vi "S4GUI_001.vi"() -> ()   [LabVIEW 2018] (continued)
                n1368 = call-dynamic "Write Channel.vi"("error in (no error)"=w2937, "Channel.lvclass"=w2938, "Acquisition in"=w2967) -> ("error out"=w2933:errorcluster, "Acquisition out"=w2934:refnum<class "Acquisition.lvclass">)  [unwired: 7 in]
              }
            }
            n1369 = case shown="True" w2918 {
              tunnel: w2920 -> [w3009 w3014]
              tunnel: w2919 -> [w3008 w3013]
              tunnel: [w3009 w3012] -> w2889
              tunnel: [w3008 w3011] -> w2888
              tunnel: w2882 -> [_ w3010]
              frame False {
              }
              frame True {
                # "nome do arquivo .cfg"
                # "seção no arquivo .cfg"
                n1370 = call-dynamic "Read Channel.vi"("error in (no error)"=w3013, "Acquisition in"=w3014) -> ("error out"=w3018:errorcluster, "Channel.lvclass"=w3017:refnum<class "Channel.lvclass">, "Acquisition out"=w3016:refnum<class "Acquisition.lvclass">)  [unwired: 7 in]
                n1371 = call-dynamic "Read Interface.vi"("error in (no error)"=w3018, "Channel in"=w3017) -> ("error out"=w3025:errorcluster, "Interface.lvclass"=w3026:refnum<class "Interface.lvclass">, "Channel out"=w3015:refnum<class "Channel.lvclass">)  [unwired: 7 in]
                n1372 = call-dynamic "Get CCD_Config.vi"("error in (no error)"=w3025, "Interface in"=w3026) -> ("error out"=w3023:errorcluster, "output cluster"=w3022:T24, "Interface out"=w3027:refnum<class "Interface.lvclass">)  [unwired: 7 in]
                n1373 = Bundle By Name(cluster=w3022, "TRIGGER_MODE"=w3010) -> (w3024:T24)
                n1374 = call-dynamic "Set CCD_Config.vi"("error in (no error)"=w3023, "input cluster"=w3024, "Interface in"=w3027) -> ("error out"=w3021:errorcluster, "Interface out"=w3028:refnum<class "Interface.lvclass">)  [unwired: 7 in]
                n1375 = Flatten To String(anything=w3024, error in (no error)=w3021) -> (data string=w3019:string, error out=w3020:errorcluster)  [unwired: 2 in, 1 out]
                n1376 = call "Write flatted cluster.vi"("error in (no error)"=w3020, "flatted cluster"=w3019, "Interface in"=w3028) -> ("error out"=w3030:errorcluster, "Interface out"=w3029:refnum<class "Interface.lvclass">)  [unwired: 7 in]
                n1377 = call-dynamic "Write Interface.vi"("error in (no error)"=w3030, "Interface.lvclass"=w3029, "Channel in"=w3015) -> ("error out"=w3036:errorcluster, "Channel out"=w3037:refnum<class "Channel.lvclass">)  [unwired: 7 in]
                n1378 = call "Write section_name.vi"("error in (no error)"=w3036, "section_name"="CCD_ACS2", "Channel in"=w3037) -> ("error out"=w3034:errorcluster, "Channel out"=w3040:refnum<class "Channel.lvclass">)  [unwired: 7 in]
                n1379 = call-dynamic "save config.vi"("error in (no error)"=w3034, "file config"="lastsaved.cfg", "Channel in"=w3040) -> ("error out"=w3035:errorcluster, "Channel out"=w3041:refnum<class "Channel.lvclass">)  [unwired: 7 in]
                n1380 = call-dynamic "Read State Machine.vi"("error in (no error)"=w3035, "Device in"=w3041) -> ("error out"=w3031:errorcluster, "State Machine.lvclass"=w3043:refnum<class "State Machine.lvclass">, "Device out"=w3042:refnum<class "Channel.lvclass">)  [unwired: 7 in]
                n1381 = call-dynamic "Write State.vi"("error in (no error)"=w3031, "State"=60, "State Machine in"=w3043) -> ("error out"=w3032:errorcluster, "State Machine out"=w3044:refnum<class "State Machine.lvclass">)  [unwired: 7 in]
                n1382 = call-dynamic "Write State Machine.vi"("error in (no error)"=w3032, "State Machine.lvclass"=w3044, "Device in"=w3042) -> ("error out"=w3046:errorcluster, "Device out"=w3045:refnum<class "Channel.lvclass">)  [unwired: 7 in]
                n1383 = call-dynamic "Write Channel.vi"("error in (no error)"=w3046, "Channel.lvclass"=w3045, "Acquisition in"=w3016) -> ("error out"=w3011:errorcluster, "Acquisition out"=w3012:refnum<class "Acquisition.lvclass">)  [unwired: 7 in]
              }
            }
            n1384 = case shown="True" w2921 {
              tunnel: [w3047 w3081] -> w2890
              tunnel: [w3048 w3080] -> w2891
              tunnel: w2923 -> [w3048 w3051]
              tunnel: w2922 -> [w3047 w3050]
              tunnel: w2882 -> [_ w3049]
              frame False {
              }
              frame True {
                # "nome do arquivo .cfg"
                # "seção no arquivo .cfg"
                n1385 = call-dynamic "Read Channel.vi"("error in (no error)"=w3050, "Acquisition in"=w3051) -> ("error out"=w3082:errorcluster, "Channel.lvclass"=w3083:refnum<class "Channel.lvclass">, "Acquisition out"=w3084:refnum<class "Acquisition.lvclass">)  [unwired: 7 in]
                n1386 = call-dynamic "Read Interface.vi"("error in (no error)"=w3082, "Channel in"=w3083) -> ("error out"=w3073:errorcluster, "Interface.lvclass"=w3072:refnum<class "Interface.lvclass">, "Channel out"=w3085:refnum<class "Channel.lvclass">)  [unwired: 7 in]
                n1387 = call-dynamic "Get CCD_Config.vi"("error in (no error)"=w3073, "Interface in"=w3072) -> ("error out"=w3075:errorcluster, "output cluster"=w3076:T24, "Interface out"=w3071:refnum<class "Interface.lvclass">)  [unwired: 7 in]
                n1388 = Bundle By Name(cluster=w3076, "TRIGGER_MODE"=w3049) -> (w3074:T24)
                n1389 = call-dynamic "Set CCD_Config.vi"("error in (no error)"=w3075, "input cluster"=w3074, "Interface in"=w3071) -> ("error out"=w3077:errorcluster, "Interface out"=w3070:refnum<class "Interface.lvclass">)  [unwired: 7 in]
                n1390 = Flatten To String(anything=w3074, error in (no error)=w3077) -> (data string=w3079:string, error out=w3078:errorcluster)  [unwired: 2 in, 1 out]
                n1391 = call "Write flatted cluster.vi"("error in (no error)"=w3078, "flatted cluster"=w3079, "Interface in"=w3070) -> ("error out"=w3068:errorcluster, "Interface out"=w3069:refnum<class "Interface.lvclass">)  [unwired: 7 in]
                n1392 = call-dynamic "Write Interface.vi"("error in (no error)"=w3068, "Interface.lvclass"=w3069, "Channel in"=w3085) -> ("error out"=w3063:errorcluster, "Channel out"=w3062:refnum<class "Channel.lvclass">)  [unwired: 7 in]
                n1393 = call "Write section_name.vi"("error in (no error)"=w3063, "section_name"="CCD_ACS1", "Channel in"=w3062) -> ("error out"=w3064:errorcluster, "Channel out"=w3059:refnum<class "Channel.lvclass">)  [unwired: 7 in]
                n1394 = call-dynamic "save config.vi"("error in (no error)"=w3064, "file config"="lastsaved.cfg", "Channel in"=w3059) -> ("error out"=w3052:errorcluster, "Channel out"=w3053:refnum<class "Channel.lvclass">)  [unwired: 7 in]
                n1395 = call-dynamic "Read State Machine.vi"("error in (no error)"=w3052, "Device in"=w3053) -> ("error out"=w3067:errorcluster, "State Machine.lvclass"=w3057:refnum<class "State Machine.lvclass">, "Device out"=w3058:refnum<class "Channel.lvclass">)  [unwired: 7 in]
                n1396 = call-dynamic "Write State.vi"("error in (no error)"=w3067, "State"=60, "State Machine in"=w3057) -> ("error out"=w3066:errorcluster, "State Machine out"=w3056:refnum<class "State Machine.lvclass">)  [unwired: 7 in]
                n1397 = call-dynamic "Write State Machine.vi"("error in (no error)"=w3066, "State Machine.lvclass"=w3056, "Device in"=w3058) -> ("error out"=w3054:errorcluster, "Device out"=w3055:refnum<class "Channel.lvclass">)  [unwired: 7 in]
                n1398 = call-dynamic "Write Channel.vi"("error in (no error)"=w3054, "Channel.lvclass"=w3055, "Acquisition in"=w3084) -> ("error out"=w3081:errorcluster, "Acquisition out"=w3080:refnum<class "Acquisition.lvclass">)  [unwired: 7 in]
              }
            }
            n1399 = call-dynamic "Write AcquisitionA.vi"("error in (no error)"=w2890, "Acquisition.lvclass"=w2891, "S4ACS_GUI in"=w2892) -> ("error out"=w2898:errorcluster, "S4ACS_GUI out"=w2901:refnum<class "S4GUI.lvclass">)  [unwired: 7 in]
            n1400 = call "Write AcquisitionB.vi"("error in (no error)"=w2888, "Acquisition.lvclass"=w2889, "S4ACS_GUI in"=w2901) -> ("error out"=w2897:errorcluster, "S4ACS_GUI out"=w2900:refnum<class "S4GUI.lvclass">)  [unwired: 7 in]
            n1401 = call-dynamic "Write AcquisitionC.vi"("error in (no error)"=w2886, "Acquisition.lvclass"=w2887, "S4ACS_GUI in"=w2900) -> ("error out"=w2896:errorcluster, "S4ACS_GUI out"=w2899:refnum<class "S4GUI.lvclass">)  [unwired: 7 in]
            n1402 = call-dynamic "Write AcquisitionD.vi"("error in (no error)"=w2884, "Acquisition.lvclass"=w2885, "S4ACS_GUI in"=w2899) -> ("error out"=w2895:errorcluster, "S4ACS_GUI out"=w2894:refnum<class "S4GUI.lvclass">)  [unwired: 7 in]
            n1403 = Merge Errors(w2898, w2897, w2896, w2895) -> (w2893:errorcluster)
          }
        }
        n1404 = call-dynamic "Write sync.vi"("error in (no error)"=w2669, "sync"=w2672, "S4ACS_GUI in"=w2670) -> ("error out"=w2658:errorcluster, "S4ACS_GUI out"=w2671:refnum<class "S4GUI.lvclass">)  [unwired: 7 in]
      }
      event "ExtSync": Value Change {
        n1405 = event-data() -> ("NewVal"=w3169:bool)  [unwired: 1 in]
        n1406 = Not(x=w3169) -> (.not. x?=w3088:bool)
        n1407 = call-dynamic "Read Sync Box.lvclass.vi"("error in (no error)"=w3172, "SPARC4_AC in"=w3181) -> ("error out"=w3174:errorcluster, "Sync Box.lvclass"=w3180:refnum<class "Sync Box.lvclass">, "SPARC4_AC out"=w3177:refnum<class "S4GUI.lvclass">)  [unwired: 7 in]
        n1408 = call-dynamic "Read Stream.vi"("error in (no error)"=w3174, "Server in"=w3180) -> ("error out"=w3173:errorcluster, "Stream.lvclass"=w3182:refnum<class "Stream.lvclass">, "Server out"=w3171:refnum<class "Sync Box.lvclass">)  [unwired: 7 in]
        n1409 = case shown="True" w3169 {
          tunnel: [w3187 w3204] -> w3175
          tunnel: w3182 -> [w3189 w3192]
          tunnel: [w3188 w3200] -> w3179
          tunnel: w3173 -> [w3185 w3191]
          tunnel: w3171 -> [w3186 w3194]
          tunnel: [w3183 w3193] -> w3170
          frame False {
            n1410 = call-dynamic "ReleaseQueueTCPIP.vi"("error in (no error)"=w3185, "Server in"=w3186) -> ("error out"=w3184:errorcluster, "Server out"=w3183:refnum<class "Sync Box.lvclass">)  [unwired: 8 in]
            n1411 = call-dynamic "End.vi"("error in (no error)"=w3184, "Stream in"=w3189) -> ("error out"=w3187:errorcluster, "Stream out"=w3188:refnum<class "Stream.lvclass">)  [unwired: 8 in]
          }
          frame True {
            w3197 = errorcluster {"status"=FALSE, "code"=0, "source"=""} ("error in (no error)")
            w3216 = FALSE ("Wait Until Done")
            w3211 = FALSE ("Wait Until Done")
            n1412 = call-dynamic "Send TCP Param.vi"("error in (no error)"=w3191, "Server in"=w3194) -> ("error out"=w3190:errorcluster, "Server out"=w3193:refnum<class "Sync Box.lvclass">)  [unwired: 8 in]
            n1413 = call-dynamic "Read StreamRX filename.vi"("error in (no error)"=w3190, "Stream in"=w3192) -> ("error out"=w3207:errorcluster, "StreamRX filename"=w3208:string, "Stream out"=w3203:refnum<class "Stream.lvclass">)  [unwired: 7 in]
            n1414 = call <vilib>:"Application Directory.vi"() -> ("Application Directory"=w3213:path)
            n1415 = call <vilib>:"Application Directory.vi"() -> ("Application Directory"=w3217:path)
            n1416 = Build Path(base path=w3217, name or relative path=w3208) -> (appended path=w3218:path)
            n1417 = Open VI Reference(vi path=w3218, error in (no error)=w3207) -> (vi reference=w3210:refnum<vi>, error out=w3209:errorcluster)  [unwired: 4 in]
            n1418 = invoke class="VI" method="Run VI"(reference=w3210, error in=w3209, "Wait until done"=w3211, "Auto Dispose Ref"=w3211) -> (reference out=w3199:refnum<vi>, error out=→"error out 7":errorcluster)  [unwired: 1 in, 3 out]
            n1419 = call-dynamic "Write stream writer vi ref.vi"("error in (no error)"=w3197, "stream writer vi ref"=w3199, "Stream in"=w3203) -> ("error out"=w3205:errorcluster, "Stream out"=w3202:refnum<class "Stream.lvclass">)  [unwired: 7 in]
            n1420 = call-dynamic "Read StreamTX filename.vi"("Stream in"=w3202) -> ("StreamTX filename"=w3206:string, "Stream out"=w3201:refnum<class "Stream.lvclass">)  [unwired: 8 in, 1 out]
            n1421 = Build Path(base path=w3213, name or relative path=w3206) -> (appended path=w3212:path)
            n1422 = Open VI Reference(vi path=w3212, error in (no error)=w3205) -> (vi reference=w3214:refnum<vi>, error out=w3215:errorcluster)  [unwired: 4 in]
            n1423 = invoke class="VI" method="Run VI"(reference=w3214, error in=w3215, "Wait until done"=w3216, "Auto Dispose Ref"=w3216) -> (reference out=w3198:refnum<vi>, error out=→"error out 8":errorcluster)  [unwired: 1 in, 3 out]
            n1424 = call-dynamic "Write stream reader vi ref.vi"("error in (no error)"=w3197, "stream reader vi ref"=w3198, "Stream in"=w3201) -> ("error out"=w3204:errorcluster, "Stream out"=w3200:refnum<class "Stream.lvclass">)  [unwired: 7 in]
          }
        }
        n1425 = call-dynamic "Write Stream.vi"("error in (no error)"=w3175, "Stream.lvclass"=w3179, "Server in"=w3170) -> ("error out"=w3176:errorcluster, "Server out"=w3178:refnum<class "Sync Box.lvclass">)  [unwired: 7 in]
        n1426 = call-dynamic "Write Sync Box.lvclass.vi"("error in (no error)"=w3176, "Sync Box.lvclass"=w3178, "SPARC4_AC in"=w3177) -> ("error out"=w3167:errorcluster, "SPARC4_AC out"=w3168:refnum<class "S4GUI.lvclass">)  [unwired: 7 in]
        n1427 = call-dynamic "Read AcquisitionC.vi"("error in (no error)"=w3167, "S4ACS_GUI in"=w3168) -> ("error out"=w3110:errorcluster, "Acquisition.lvclass"=w3111:refnum<class "Acquisition.lvclass">)  [unwired: 7 in, 1 out]
        n1428 = call-dynamic "Read AcquisitionA.vi"("error in (no error)"=w3167, "S4ACS_GUI in"=w3168) -> ("error out"=w3147:errorcluster, "Acquisition.lvclass"=w3146:refnum<class "Acquisition.lvclass">, "S4ACS_GUI out"=w3163:refnum<class "S4GUI.lvclass">)  [unwired: 7 in]
        n1429 = call "Read AcquisitionB.vi"("error in (no error)"=w3167, "S4ACS_GUI in"=w3168) -> ("error out"=w3127:errorcluster, "Acquisition.lvclass"=w3128:refnum<class "Acquisition.lvclass">)  [unwired: 7 in, 1 out]
        n1430 = call-dynamic "Read AcquisitionD.vi"("error in (no error)"=w3167, "S4ACS_GUI in"=w3168) -> ("error out"=w3093:errorcluster, "Acquisition.lvclass"=w3094:refnum<class "Acquisition.lvclass">)  [unwired: 7 in, 1 out]
        n1431 = call-dynamic "Read Channel.vi"("error in (no error)"=w3093, "Acquisition in"=w3094) -> ("error out"=w3096:errorcluster, "Channel.lvclass"=w3098:refnum<class "Channel.lvclass">, "Acquisition out"=w3107:refnum<class "Acquisition.lvclass">)  [unwired: 7 in]
        n1432 = call-dynamic "Read Channel.vi"("error in (no error)"=w3110, "Acquisition in"=w3111) -> ("error out"=w3113:errorcluster, "Channel.lvclass"=w3115:refnum<class "Channel.lvclass">, "Acquisition out"=w3124:refnum<class "Acquisition.lvclass">)  [unwired: 7 in]
        n1433 = call-dynamic "Read Channel.vi"("error in (no error)"=w3127, "Acquisition in"=w3128) -> ("error out"=w3130:errorcluster, "Channel.lvclass"=w3132:refnum<class "Channel.lvclass">, "Acquisition out"=w3141:refnum<class "Acquisition.lvclass">)  [unwired: 7 in]
        n1434 = call-dynamic "Read Channel.vi"("error in (no error)"=w3147, "Acquisition in"=w3146) -> ("error out"=w3143:errorcluster, "Channel.lvclass"=w3145:refnum<class "Channel.lvclass">, "Acquisition out"=w3156:refnum<class "Acquisition.lvclass">)  [unwired: 7 in]
        n1435 = call-dynamic "Write wait_expose.vi"("error in (no error)"=w3096, "wait_expose"=w3088, "Channel in"=w3098) -> ("error out"=w3095:errorcluster, "Channel out"=w3097:refnum<class "Channel.lvclass">)  [unwired: 7 in]
        n1436 = call-dynamic "Write wait_expose.vi"("error in (no error)"=w3113, "wait_expose"=w3088, "Channel in"=w3115) -> ("error out"=w3112:errorcluster, "Channel out"=w3114:refnum<class "Channel.lvclass">)  [unwired: 7 in]
        n1437 = call-dynamic "Write wait_expose.vi"("error in (no error)"=w3130, "wait_expose"=w3088, "Channel in"=w3132) -> ("error out"=w3129:errorcluster, "Channel out"=w3131:refnum<class "Channel.lvclass">)  [unwired: 7 in]
        n1438 = call-dynamic "Write wait_expose.vi"("error in (no error)"=w3143, "wait_expose"=w3088, "Channel in"=w3145) -> ("error out"=w3142:errorcluster, "Channel out"=w3144:refnum<class "Channel.lvclass">)  [unwired: 7 in]
        n1439 = call-dynamic "Read State Machine.vi"("error in (no error)"=w3095, "Device in"=w3097) -> ("error out"=w3106:errorcluster, "State Machine.lvclass"=w3102:refnum<class "State Machine.lvclass">, "Device out"=w3103:refnum<class "Channel.lvclass">)  [unwired: 7 in]
        n1440 = call-dynamic "Read State Machine.vi"("error in (no error)"=w3112, "Device in"=w3114) -> ("error out"=w3123:errorcluster, "State Machine.lvclass"=w3119:refnum<class "State Machine.lvclass">, "Device out"=w3120:refnum<class "Channel.lvclass">)  [unwired: 7 in]
        n1441 = call-dynamic "Read State Machine.vi"("error in (no error)"=w3129, "Device in"=w3131) -> ("error out"=w3140:errorcluster, "State Machine.lvclass"=w3136:refnum<class "State Machine.lvclass">, "Device out"=w3137:refnum<class "Channel.lvclass">)  [unwired: 7 in]
        n1442 = call-dynamic "Read State Machine.vi"("error in (no error)"=w3142, "Device in"=w3144) -> ("error out"=w3155:errorcluster, "State Machine.lvclass"=w3151:refnum<class "State Machine.lvclass">, "Device out"=w3152:refnum<class "Channel.lvclass">)  [unwired: 7 in]
        n1443 = call-dynamic "Write State.vi"("error in (no error)"=w3106, "State"=40, "State Machine in"=w3102) -> ("error out"=w3105:errorcluster, "State Machine out"=w3101:refnum<class "State Machine.lvclass">)  [unwired: 7 in]
        n1444 = call-dynamic "Write State.vi"("error in (no error)"=w3123, "State"=40, "State Machine in"=w3119) -> ("error out"=w3122:errorcluster, "State Machine out"=w3118:refnum<class "State Machine.lvclass">)  [unwired: 7 in]
        n1445 = call-dynamic "Write State.vi"("error in (no error)"=w3140, "State"=40, "State Machine in"=w3136) -> ("error out"=w3139:errorcluster, "State Machine out"=w3135:refnum<class "State Machine.lvclass">)  [unwired: 7 in]
        n1446 = call-dynamic "Write State.vi"("error in (no error)"=w3155, "State"=40, "State Machine in"=w3151) -> ("error out"=w3154:errorcluster, "State Machine out"=w3150:refnum<class "State Machine.lvclass">)  [unwired: 7 in]
        n1447 = call-dynamic "Write State Machine.vi"("error in (no error)"=w3105, "State Machine.lvclass"=w3101, "Device in"=w3103) -> ("error out"=w3099:errorcluster, "Device out"=w3100:refnum<class "Channel.lvclass">)  [unwired: 7 in]
        n1448 = call-dynamic "Write State Machine.vi"("error in (no error)"=w3122, "State Machine.lvclass"=w3118, "Device in"=w3120) -> ("error out"=w3116:errorcluster, "Device out"=w3117:refnum<class "Channel.lvclass">)  [unwired: 7 in]
        n1449 = call-dynamic "Write State Machine.vi"("error in (no error)"=w3139, "State Machine.lvclass"=w3135, "Device in"=w3137) -> ("error out"=w3133:errorcluster, "Device out"=w3134:refnum<class "Channel.lvclass">)  [unwired: 7 in]
        n1450 = call-dynamic "Write State Machine.vi"("error in (no error)"=w3154, "State Machine.lvclass"=w3150, "Device in"=w3152) -> ("error out"=w3148:errorcluster, "Device out"=w3149:refnum<class "Channel.lvclass">)  [unwired: 7 in]
        n1451 = call-dynamic "Write Channel.vi"("error in (no error)"=w3099, "Channel.lvclass"=w3100, "Acquisition in"=w3107) -> ("error out"=w3091:errorcluster, "Acquisition out"=w3092:refnum<class "Acquisition.lvclass">)  [unwired: 7 in]
        n1452 = call-dynamic "Write Channel.vi"("error in (no error)"=w3116, "Channel.lvclass"=w3117, "Acquisition in"=w3124) -> ("error out"=w3109:errorcluster, "Acquisition out"=w3108:refnum<class "Acquisition.lvclass">)  [unwired: 7 in]
        n1453 = call-dynamic "Write Channel.vi"("error in (no error)"=w3133, "Channel.lvclass"=w3134, "Acquisition in"=w3141) -> ("error out"=w3126:errorcluster, "Acquisition out"=w3125:refnum<class "Acquisition.lvclass">)  [unwired: 7 in]
        n1454 = call-dynamic "Write Channel.vi"("error in (no error)"=w3148, "Channel.lvclass"=w3149, "Acquisition in"=w3156) -> ("error out"=w3161:errorcluster, "Acquisition out"=w3162:refnum<class "Acquisition.lvclass">)  [unwired: 7 in]
        n1455 = call-dynamic "Write AcquisitionA.vi"("error in (no error)"=w3161, "Acquisition.lvclass"=w3162, "S4ACS_GUI in"=w3163) -> ("error out"=w3160:errorcluster, "S4ACS_GUI out"=w3166:refnum<class "S4GUI.lvclass">)  [unwired: 7 in]
        n1456 = call "Write AcquisitionB.vi"("error in (no error)"=w3126, "Acquisition.lvclass"=w3125, "S4ACS_GUI in"=w3166) -> ("error out"=w3159:errorcluster, "S4ACS_GUI out"=w3165:refnum<class "S4GUI.lvclass">)  [unwired: 7 in]
        n1457 = call-dynamic "Write AcquisitionC.vi"("error in (no error)"=w3109, "Acquisition.lvclass"=w3108, "S4ACS_GUI in"=w3165) -> ("error out"=w3158:errorcluster, "S4ACS_GUI out"=w3164:refnum<class "S4GUI.lvclass">)  [unwired: 7 in]
        n1458 = call-dynamic "Write AcquisitionD.vi"("error in (no error)"=w3091, "Acquisition.lvclass"=w3092, "S4ACS_GUI in"=w3164) -> ("error out"=w3157:errorcluster, "S4ACS_GUI out"=w3090:refnum<class "S4GUI.lvclass">)  [unwired: 7 in]
        n1459 = Merge Errors(w3160, w3159, w3158, w3157) -> (w3089:errorcluster)
        n1460 = call-dynamic "Write mode EXPOSE.vi"("error in (no error)"=w3089, "mode EXPOSE"=w3088, "S4GUI in"=w3090) -> ("error out"=w3086:errorcluster, "S4GUI out"=w3087:refnum<class "S4GUI.lvclass">)  [unwired: 7 in]
      }
      event "Run WPROT": Value Change {
        n1461 = event-data() -> ("NewVal"=w3226:bool)  [unwired: 1 in]
        n1462 = case shown="True" w3226 {
          tunnel: [u32 0 ("Ciclos  WPROT") "Ciclos  WPROT"] -> w3225
          tunnel: w3222 -> [w3228 w3233]
          tunnel: [w3228 w3232] -> w3221
          tunnel: w3220 -> [w3227 w3231]
          tunnel: [w3227 w3230] -> w3219
          frame False {
          }
          frame True {
            n1463 = call-dynamic "Write Obs_state.vi"("error in (no error)"=w3231, "Obs_state"=u32 350, "S4ACS_GUI in"=w3233) -> ("error out"=w3230:errorcluster, "S4ACS_GUI out"=w3232:refnum<class "S4GUI.lvclass">)  [unwired: 7 in]
          }
        }
        n1464 = call-dynamic "Write cycles wprot.vi"("error in (no error)"=w3219, "cycles wprot"=w3225, "S4GUI in"=w3221) -> ("error out"=w3223:errorcluster, "S4GUI out"=w3224:refnum<class "S4GUI.lvclass">)  [unwired: 7 in]
      }
      event "Start SM": Value Change {
        n1465 = event-data() -> ()  [unwired: 1 in, 6 out]
        n1466 = call-dynamic "Read Obs_state.vi"("error in (no error)"=w3256, "S4ACS_GUI in"=w3257) -> ("error out"=w3241:errorcluster, "Obs_state"=w3254:u32, "S4ACS_GUI out"=w3243:refnum<class "S4GUI.lvclass">)  [unwired: 7 in]
        n1467 = call "Read Instrument.lvclass.vi"("error in (no error)"=w3241, "S4ACS_GUI in"=w3243) -> ("error out"=w3239:errorcluster, "Instrument.lvclass"=w3240:refnum<class "Instrument.lvclass">, "S4ACS_GUI out"=w3242:refnum<class "S4GUI.lvclass">)  [unwired: 7 in]
        n1468 = Not Equal?(x=w3254, y=u32 400) -> (x != y?=w3253:bool)
        n1469 = call-dynamic "Read mode.vi"("error in (no error)"=w3239, "Instrument in"=w3240) -> ("error out"=w3238:errorcluster, "mode"=w3237:bool)  [unwired: 7 in, 1 out]
        n1470 = case shown="True" w3253 {
          tunnel: w3242 -> [w3324 w3378]
          tunnel: w3238 -> [w3320 w3376]
          tunnel: [w3259 w3391] -> w3247
          tunnel: [w3258 w3389] -> w3251
          tunnel: w3249 -> [_ w3398]
          tunnel: w3248 -> [_ w3397]
          tunnel: w3246 -> [_ w3396]
          tunnel: w3245 -> [_ w3395]
          tunnel: w3244 -> [_ w3394]
          tunnel: w3237 -> [_ w3393]
          tunnel: w3236 -> [_ w3373]
          frame False {
            # "Obs_state=400 (PAUSED), então retoma a execução do estado onde parou."
            n1471 = call-dynamic "Read Obs_prevstate.vi"("error in (no error)"=w3320, "S4ACS_GUI in"=w3324) -> ("error out"=w3321:errorcluster, "Obs_prevstate"=w3323:u32, "S4ACS_GUI out"=w3322:refnum<class "S4GUI.lvclass">)  [unwired: 7 in]
            n1472 = call-dynamic "Write Obs_state.vi"("error in (no error)"=w3321, "Obs_state"=w3323, "S4ACS_GUI in"=w3322) -> ("error out"=w3260:errorcluster, "S4ACS_GUI out"=w3261:refnum<class "S4GUI.lvclass">)  [unwired: 7 in]
            n1473 = call-dynamic "Read AcquisitionA.vi"("error in (no error)"=w3260, "S4ACS_GUI in"=w3261) -> ("error out"=w3314:errorcluster, "Acquisition.lvclass"=w3318:refnum<class "Acquisition.lvclass">, "S4ACS_GUI out"=w3319:refnum<class "S4GUI.lvclass">)  [unwired: 7 in]
            n1474 = call-dynamic "Read Channel.vi"("error in (no error)"=w3314, "Acquisition in"=w3318) -> ("error out"=w3285:errorcluster, "Channel.lvclass"=w3286:refnum<class "Channel.lvclass">, "Acquisition out"=w3317:refnum<class "Acquisition.lvclass">)  [unwired: 7 in]
            n1475 = call "Read connected.vi"("error in (no error)"=w3285, "Device in"=w3286) -> ("error out"=w3284:errorcluster, "connected"=w3283:bool, "Device out"=w3287:refnum<class "Channel.lvclass">)  [unwired: 7 in]
            n1476 = case shown="True" w3283 {
              tunnel: w3287 -> [w3362 w3372]
              tunnel: [w3362 w3370] -> w3315
              tunnel: w3284 -> [w3361 w3367]
              tunnel: [w3361 w3365] -> w3313
              frame False {
              }
              frame True {
                n1477 = call-dynamic "Read State Machine.vi"("error in (no error)"=w3367, "Device in"=w3372) -> ("error out"=w3363:errorcluster, "State Machine.lvclass"=w3364:refnum<class "State Machine.lvclass">, "Device out"=w3371:refnum<class "Channel.lvclass">)  [unwired: 7 in]
                n1478 = call "Next State.vi"("error in (no error)"=w3363, "New_State"=96, "State Machine in"=w3364) -> ("error out"=w3366:errorcluster, "State Machine out"=w3369:refnum<class "State Machine.lvclass">)  [unwired: 7 in]
                n1479 = call-dynamic "Write State Machine.vi"("error in (no error)"=w3366, "State Machine.lvclass"=w3369, "Device in"=w3371) -> ("error out"=w3365:errorcluster, "Device out"=w3370:refnum<class "Channel.lvclass">)  [unwired: 7 in]
              }
            }
            n1480 = call-dynamic "Write Channel.vi"("error in (no error)"=w3313, "Channel.lvclass"=w3315, "Acquisition in"=w3317) -> ("error out"=w3312:errorcluster, "Acquisition out"=w3316:refnum<class "Acquisition.lvclass">)  [unwired: 7 in]
            n1481 = call-dynamic "Write AcquisitionA.vi"("error in (no error)"=w3312, "Acquisition.lvclass"=w3316, "S4ACS_GUI in"=w3319) -> ("error out"=w3293:errorcluster, "S4ACS_GUI out"=w3290:refnum<class "S4GUI.lvclass">)  [unwired: 7 in]
            n1482 = call "Read AcquisitionB.vi"("error in (no error)"=w3293, "S4ACS_GUI in"=w3290) -> ("error out"=w3307:errorcluster, "Acquisition.lvclass"=w3310:refnum<class "Acquisition.lvclass">, "S4ACS_GUI out"=w3311:refnum<class "S4GUI.lvclass">)  [unwired: 7 in]
            n1483 = call-dynamic "Read Channel.vi"("error in (no error)"=w3307, "Acquisition in"=w3310) -> ("error out"=w3278:errorcluster, "Channel.lvclass"=w3279:refnum<class "Channel.lvclass">, "Acquisition out"=w3309:refnum<class "Acquisition.lvclass">)  [unwired: 7 in]
            n1484 = call "Read connected.vi"("error in (no error)"=w3278, "Device in"=w3279) -> ("error out"=w3281:errorcluster, "connected"=w3280:bool, "Device out"=w3282:refnum<class "Channel.lvclass">)  [unwired: 7 in]
            n1485 = case shown="True" w3280 {
              tunnel: w3282 -> [w3350 w3360]
              tunnel: [w3350 w3358] -> w3276
              tunnel: w3281 -> [w3349 w3355]
              tunnel: [w3349 w3353] -> w3277
              frame False {
              }
              frame True {
                n1486 = call-dynamic "Read State Machine.vi"("error in (no error)"=w3355, "Device in"=w3360) -> ("error out"=w3351:errorcluster, "State Machine.lvclass"=w3352:refnum<class "State Machine.lvclass">, "Device out"=w3359:refnum<class "Channel.lvclass">)  [unwired: 7 in]
                n1487 = call "Next State.vi"("error in (no error)"=w3351, "New_State"=96, "State Machine in"=w3352) -> ("error out"=w3354:errorcluster, "State Machine out"=w3357:refnum<class "State Machine.lvclass">)  [unwired: 7 in]
                n1488 = call-dynamic "Write State Machine.vi"("error in (no error)"=w3354, "State Machine.lvclass"=w3357, "Device in"=w3359) -> ("error out"=w3353:errorcluster, "Device out"=w3358:refnum<class "Channel.lvclass">)  [unwired: 7 in]
              }
            }
            n1489 = call-dynamic "Write Channel.vi"("error in (no error)"=w3277, "Channel.lvclass"=w3276, "Acquisition in"=w3309) -> ("error out"=w3306:errorcluster, "Acquisition out"=w3308:refnum<class "Acquisition.lvclass">)  [unwired: 7 in]
            n1490 = call "Write AcquisitionB.vi"("error in (no error)"=w3306, "Acquisition.lvclass"=w3308, "S4ACS_GUI in"=w3311) -> ("error out"=w3292:errorcluster, "S4ACS_GUI out"=w3289:refnum<class "S4GUI.lvclass">)  [unwired: 7 in]
            n1491 = call-dynamic "Read AcquisitionC.vi"("error in (no error)"=w3292, "S4ACS_GUI in"=w3289) -> ("error out"=w3301:errorcluster, "Acquisition.lvclass"=w3304:refnum<class "Acquisition.lvclass">, "S4ACS_GUI out"=w3305:refnum<class "S4GUI.lvclass">)  [unwired: 7 in]
            n1492 = call-dynamic "Read Channel.vi"("error in (no error)"=w3301, "Acquisition in"=w3304) -> ("error out"=w3271:errorcluster, "Channel.lvclass"=w3272:refnum<class "Channel.lvclass">, "Acquisition out"=w3303:refnum<class "Acquisition.lvclass">)  [unwired: 7 in]
            n1493 = call "Read connected.vi"("error in (no error)"=w3271, "Device in"=w3272) -> ("error out"=w3274:errorcluster, "connected"=w3273:bool, "Device out"=w3275:refnum<class "Channel.lvclass">)  [unwired: 7 in]
            n1494 = case shown="True" w3273 {
              tunnel: w3275 -> [w3338 w3348]
              tunnel: [w3338 w3346] -> w3270
              tunnel: w3274 -> [w3337 w3343]
              tunnel: [w3337 w3341] -> w3269
              frame False {
              }
              frame True {
                n1495 = call-dynamic "Read State Machine.vi"("error in (no error)"=w3343, "Device in"=w3348) -> ("error out"=w3339:errorcluster, "State Machine.lvclass"=w3340:refnum<class "State Machine.lvclass">, "Device out"=w3347:refnum<class "Channel.lvclass">)  [unwired: 7 in]
                n1496 = call "Next State.vi"("error in (no error)"=w3339, "New_State"=96, "State Machine in"=w3340) -> ("error out"=w3342:errorcluster, "State Machine out"=w3345:refnum<class "State Machine.lvclass">)  [unwired: 7 in]
                n1497 = call-dynamic "Write State Machine.vi"("error in (no error)"=w3342, "State Machine.lvclass"=w3345, "Device in"=w3347) -> ("error out"=w3341:errorcluster, "Device out"=w3346:refnum<class "Channel.lvclass">)  [unwired: 7 in]
              }
            }
            n1498 = call-dynamic "Write Channel.vi"("error in (no error)"=w3269, "Channel.lvclass"=w3270, "Acquisition in"=w3303) -> ("error out"=w3300:errorcluster, "Acquisition out"=w3302:refnum<class "Acquisition.lvclass">)  [unwired: 7 in]
            n1499 = call-dynamic "Write AcquisitionC.vi"("error in (no error)"=w3300, "Acquisition.lvclass"=w3302, "S4ACS_GUI in"=w3305) -> ("error out"=w3291:errorcluster, "S4ACS_GUI out"=w3288:refnum<class "S4GUI.lvclass">)  [unwired: 7 in]
            n1500 = call-dynamic "Read AcquisitionD.vi"("error in (no error)"=w3291, "S4ACS_GUI in"=w3288) -> ("error out"=w3295:errorcluster, "Acquisition.lvclass"=w3298:refnum<class "Acquisition.lvclass">, "S4ACS_GUI out"=w3299:refnum<class "S4GUI.lvclass">)  [unwired: 7 in]
            n1501 = call-dynamic "Read Channel.vi"("error in (no error)"=w3295, "Acquisition in"=w3298) -> ("error out"=w3264:errorcluster, "Channel.lvclass"=w3265:refnum<class "Channel.lvclass">, "Acquisition out"=w3297:refnum<class "Acquisition.lvclass">)  [unwired: 7 in]
            n1502 = call "Read connected.vi"("error in (no error)"=w3264, "Device in"=w3265) -> ("error out"=w3267:errorcluster, "connected"=w3266:bool, "Device out"=w3268:refnum<class "Channel.lvclass">)  [unwired: 7 in]
            n1503 = case shown="True" w3266 {
              tunnel: w3268 -> [w3326 w3336]
              tunnel: [w3326 w3334] -> w3263
              tunnel: w3267 -> [w3325 w3331]
              tunnel: [w3325 w3329] -> w3262
              frame False {
              }
              frame True {
                n1504 = call-dynamic "Read State Machine.vi"("error in (no error)"=w3331, "Device in"=w3336) -> ("error out"=w3327:errorcluster, "State Machine.lvclass"=w3328:refnum<class "State Machine.lvclass">, "Device out"=w3335:refnum<class "Channel.lvclass">)  [unwired: 7 in]
                n1505 = call "Next State.vi"("error in (no error)"=w3327, "New_State"=96, "State Machine in"=w3328) -> ("error out"=w3330:errorcluster, "State Machine out"=w3333:refnum<class "State Machine.lvclass">)  [unwired: 7 in]
                n1506 = call-dynamic "Write State Machine.vi"("error in (no error)"=w3330, "State Machine.lvclass"=w3333, "Device in"=w3335) -> ("error out"=w3329:errorcluster, "Device out"=w3334:refnum<class "Channel.lvclass">)  [unwired: 7 in]
              }
            }
            n1507 = call-dynamic "Write Channel.vi"("error in (no error)"=w3262, "Channel.lvclass"=w3263, "Acquisition in"=w3297) -> ("error out"=w3294:errorcluster, "Acquisition out"=w3296:refnum<class "Acquisition.lvclass">)  [unwired: 7 in]
            n1508 = call-dynamic "Write AcquisitionD.vi"("error in (no error)"=w3294, "Acquisition.lvclass"=w3296, "S4ACS_GUI in"=w3299) -> ("error out"=w3258:errorcluster, "S4ACS_GUI out"=w3259:refnum<class "S4GUI.lvclass">)  [unwired: 7 in]
          }
          frame True {
            # "aba atual em Tab Acq Type"
            n1509 = call "Read Instrument.lvclass.vi"("error in (no error)"=w3376, "S4ACS_GUI in"=w3378) -> ("error out"=w3380:errorcluster, "Instrument.lvclass"=w3382:refnum<class "Instrument.lvclass">, "S4ACS_GUI out"=w3377:refnum<class "S4GUI.lvclass">)  [unwired: 7 in]
            n1510 = call "Read WPROT.vi"("error in (no error)"=w3380, "Instrument in"=w3382) -> ("error out"=w3379:errorcluster, "Opt_Selector.lvclass"=w3381:refnum<class "Opt_Selector.lvclass">)  [unwired: 7 in, 1 out]
            n1511 = call-dynamic "Read sequencia.vi"("error in (no error)"=w3379, "Opt_Selector in"=w3381) -> ("error out"=w3375:errorcluster, "sequencia"=w3374:u16)  [unwired: 7 in, 1 out]
            n1512 = case shown="True" w3393 {
              tunnel: [0 w3405] -> w3383
              tunnel: w3374 -> [_ w3404]
              frame False {
                # "OV 20230424: \n#SEQ agora armazena as\nposições da lâmina utilizadas.\nNa fotometria, #SEQ=0"
                # "fotometria:"
              }
              frame True {
                # "polarimetria:"
                n1513 = disable-structure shown="Enabled" {
                  disable-tunnel: [w3406 w3408] -> w3405
                  disable-tunnel: w3404 -> [_ w3409]
                  frame Disabled {
                    n1514 = property on="#Polarimetric Sequence Done" class="Slide (strict)"() -> ("Scale.Maximum"=w3407:dbl)  [unwired: 2 in, 2 out]
                    n1515 = To Unsigned Long Integer(number=w3407) -> (unsigned 32bit integer=w3406:u32)
                  }
                  frame Enabled {
                    # "OV 20230424: \n#SEQ agora armazena as\nposições da lâmina utilizadas.\nNa polarimetria, #SEQ=WPROT.sequencia"
                    n1516 = To Unsigned Long Integer(number=w3409) -> (unsigned 32bit integer=w3408:u32)
                  }
                }
              }
            }
            n1517 = call-dynamic "Write Obs_state.vi"("error in (no error)"=w3375, "Obs_state"=u32 251, "S4ACS_GUI in"=w3377) -> ("error out"=w3401:errorcluster, "S4ACS_GUI out"=w3400:refnum<class "S4GUI.lvclass">)  [unwired: 7 in]
            n1518 = local read "# Cycles"() -> (w3388:u32)
            n1519 = stacked-sequence {
              seq-local: [w3434 _ _ _] -> [_ w3520 _ _]
              seq-local: [w3433 _ _ _] -> [_ w3519 _ _]
              seq-local: [_ w3518 _ _] -> [_ _ w3579 _]
              seq-local: [_ w3517 _ _] -> [_ _ w3578 _]
              seq-local: [_ _ w3577 _] -> [_ _ _ w3638]
              seq-local: [_ _ w3576 _] -> [_ _ _ w3637]
              tunnel: w3401 -> [w3454 _ _ _]
              tunnel: w3400 -> [w3453 _ _ _]
              tunnel: [_ _ _ w3636] -> w3385
              tunnel: [_ _ _ w3635] -> w3387
              tunnel: w3398 -> [w3432 w3516 w3575 w3634]
              tunnel: w3397 -> [w3431 w3515 w3549 w3608]
              tunnel: w3396 -> [w3430 w3489 w3548 w3607]
              tunnel: w3395 -> [w3429 w3488 w3547 w3606]
              tunnel: w3394 -> [w3424 w3483 w3542 w3601]
              tunnel: w3388 -> [w3421 w3480 w3539 w3598]
              tunnel: w3383 -> [w3416 w3475 w3534 w3593]
              tunnel: w3373 -> [w3410 w3471 w3530 w3587]
              frame #0 {
                # "object"
                # "suffix"
                # "obsType"
                n1520 = local read "Exptime ch1"() -> (w3411:dbl)
                n1521 = call-dynamic "Read AcquisitionA.vi"("error in (no error)"=w3454, "S4ACS_GUI in"=w3453) -> ("error out"=w3452:errorcluster, "Acquisition.lvclass"=w3451:refnum<class "Acquisition.lvclass">, "S4ACS_GUI out"=w3441:refnum<class "S4GUI.lvclass">)  [unwired: 7 in]
                n1522 = call-dynamic "Read Channel.vi"("error in (no error)"=w3452, "Acquisition in"=w3451) -> ("error out"=w3449:errorcluster, "Channel.lvclass"=w3450:refnum<class "Channel.lvclass">, "Acquisition out"=w3440:refnum<class "Acquisition.lvclass">)  [unwired: 7 in]
                n1523 = local read "Exp ch1"() -> (w3436:u32)
                n1524 = call-dynamic "Read Interface.vi"("error in (no error)"=w3449, "Channel in"=w3450) -> ("error out"=w3461:errorcluster, "Interface.lvclass"=w3447:refnum<class "Interface.lvclass">, "Channel out"=w3448:refnum<class "Channel.lvclass">)  [unwired: 7 in]
                n1525 = call "Write Exposure Time.vi"("error in (no error)"=w3461, "Exposure Time"=w3411, "Interface in"=w3447) -> ("error out"=w3412:errorcluster, "Interface out"=w3415:refnum<class "Interface.lvclass">)  [unwired: 7 in]
                n1526 = case shown="Default" w3410 {
                  tunnel: w3415 -> [w3463 w3468]
                  tunnel: [w3463 w3467] -> w3414
                  tunnel: [w3462 w3466] -> w3413
                  tunnel: w3412 -> [w3462 w3465]
                  tunnel: w3411 -> [_ w3464]
                  frame "ZERO" {
                  }
                  frame Default {
                    n1527 = call-dynamic "Write prev ExpTime.vi"("error in (no error)"=w3465, "prev ExpTime"=w3464, "Interface in"=w3468) -> ("error out"=w3466:errorcluster, "Interface out"=w3467:refnum<class "Interface.lvclass">)  [unwired: 7 in]
                  }
                }
                n1528 = call-dynamic "Write Suffix.vi"("error in (no error)"=w3413, "Suffix"=w3432, "Interface in"=w3414) -> ("error out"=w3460:errorcluster, "Interface out"=w3446:refnum<class "Interface.lvclass">)  [unwired: 7 in]
                n1529 = call-dynamic "Write ObsType.vi"("error in (no error)"=w3460, "ObsType"=w3430, "Interface in"=w3446) -> ("error out"=w3459:errorcluster, "Interface out"=w3445:refnum<class "Interface.lvclass">)  [unwired: 7 in]
                n1530 = call-dynamic "Write Object.vi"("error in (no error)"=w3459, "Object"=w3429, "Interface in"=w3445) -> ("error out"=w3458:errorcluster, "Interface out"=w3444:refnum<class "Interface.lvclass">)  [unwired: 7 in]
                n1531 = call-dynamic "Write Comments.vi"("error in (no error)"=w3458, "Comments"=w3431, "Interface in"=w3444) -> ("error out"=w3457:errorcluster, "Interface out"=w3443:refnum<class "Interface.lvclass">)  [unwired: 7 in]
                n1532 = call-dynamic "Write DS9.vi"("error in (no error)"=w3457, "DS9"="F", "Interface in"=w3443) -> ("error out"=w3426:errorcluster, "Interface out"=w3428:refnum<class "Interface.lvclass">)  [unwired: 7 in]
                n1533 = call-dynamic "Write Observer.vi"("error in (no error)"=w3426, "Observer"=w3424, "Interface in"=w3428) -> ("error out"=w3425:errorcluster, "Interface out"=w3427:refnum<class "Interface.lvclass">)  [unwired: 7 in]
                n1534 = call-dynamic "Write # Images.vi"("error in (no error)"=w3425, "# Images"=w3436, "Interface in"=w3427) -> ("error out"=w3455:errorcluster, "Interface out"=w3442:refnum<class "Interface.lvclass">)  [unwired: 7 in]
                n1535 = property on="Exposure Done ch1" class="Slide (strict)"("Scale.Maximum"=w3436, "Scale.Minimum"=0.0 ("Scale.Range:Minimum")) -> ()  [unwired: 2 in, 2 out]
                n1536 = property on="Exposure Time ch1" class="Slide (strict)"("Scale.Maximum"=w3411, "Scale.Minimum"=0.0 ("Scale.Range:Minimum")) -> ()  [unwired: 2 in, 2 out]
                n1537 = call-dynamic "Write Interface.vi"("error in (no error)"=w3455, "Interface.lvclass"=w3442, "Channel in"=w3448) -> ("error out"=w3423:errorcluster, "Channel out"=w3422:refnum<class "Channel.lvclass">)  [unwired: 7 in]
                n1538 = call-dynamic "Write ciclos.vi"("error in (no error)"=w3423, "ciclos"=w3421, "Channel in"=w3422) -> ("error out"=w3418:errorcluster, "Channel out"=w3420:refnum<class "Channel.lvclass">)  [unwired: 7 in]
                n1539 = call-dynamic "Write sequencias.vi"("error in (no error)"=w3418, "sequencias"=w3416, "Channel in"=w3420) -> ("error out"=w3417:errorcluster, "Channel out"=w3419:refnum<class "Channel.lvclass">)  [unwired: 7 in]
                n1540 = call-dynamic "Write Channel.vi"("error in (no error)"=w3417, "Channel.lvclass"=w3419, "Acquisition in"=w3440) -> ("error out"=w3438:errorcluster, "Acquisition out"=w3439:refnum<class "Acquisition.lvclass">)  [unwired: 7 in]
                n1541 = call-dynamic "Write AcquisitionA.vi"("error in (no error)"=w3438, "Acquisition.lvclass"=w3439, "S4ACS_GUI in"=w3441) -> ("error out"=w3433:errorcluster, "S4ACS_GUI out"=w3434:refnum<class "S4GUI.lvclass">)  [unwired: 7 in]
              }
              frame #1 {
                # "object"
                # "suffix"
                # "obsType"
                n1542 = call "Read AcquisitionB.vi"("error in (no error)"=w3519, "S4ACS_GUI in"=w3520) -> ("error out"=w3500:errorcluster, "Acquisition.lvclass"=w3501:refnum<class "Acquisition.lvclass">, "S4ACS_GUI out"=w3511:refnum<class "S4GUI.lvclass">)  [unwired: 7 in]
                n1543 = local read "Exptime ch2"() -> (w3472:dbl)
                n1544 = call-dynamic "Read Channel.vi"("error in (no error)"=w3500, "Acquisition in"=w3501) -> ("error out"=w3503:errorcluster, "Channel.lvclass"=w3502:refnum<class "Channel.lvclass">, "Acquisition out"=w3512:refnum<class "Acquisition.lvclass">)  [unwired: 7 in]
                n1545 = call-dynamic "Read Interface.vi"("error in (no error)"=w3503, "Channel in"=w3502) -> ("error out"=w3494:errorcluster, "Interface.lvclass"=w3505:refnum<class "Interface.lvclass">, "Channel out"=w3504:refnum<class "Channel.lvclass">)  [unwired: 7 in]
                n1546 = call "Write Exposure Time.vi"("error in (no error)"=w3494, "Exposure Time"=w3472, "Interface in"=w3505) -> ("error out"=w3473:errorcluster, "Interface out"=w3474:refnum<class "Interface.lvclass">)  [unwired: 7 in]
                n1547 = case shown="Default" w3471 {
                  tunnel: w3474 -> [w3522 w3527]
                  tunnel: [w3522 w3526] -> w3470
                  tunnel: [w3521 w3525] -> w3469
                  tunnel: w3473 -> [w3521 w3524]
                  tunnel: w3472 -> [_ w3523]
                  frame "ZERO" {
                  }
                  frame Default {
                    n1548 = call-dynamic "Write prev ExpTime.vi"("error in (no error)"=w3524, "prev ExpTime"=w3523, "Interface in"=w3527) -> ("error out"=w3525:errorcluster, "Interface out"=w3526:refnum<class "Interface.lvclass">)  [unwired: 7 in]
                  }
                }
                n1549 = call-dynamic "Write Suffix.vi"("error in (no error)"=w3469, "Suffix"=w3516, "Interface in"=w3470) -> ("error out"=w3495:errorcluster, "Interface out"=w3506:refnum<class "Interface.lvclass">)  [unwired: 7 in]
                n1550 = call-dynamic "Write ObsType.vi"("error in (no error)"=w3495, "ObsType"=w3489, "Interface in"=w3506) -> ("error out"=w3496:errorcluster, "Interface out"=w3507:refnum<class "Interface.lvclass">)  [unwired: 7 in]
                n1551 = call-dynamic "Write Object.vi"("error in (no error)"=w3496, "Object"=w3488, "Interface in"=w3507) -> ("error out"=w3497:errorcluster, "Interface out"=w3508:refnum<class "Interface.lvclass">)  [unwired: 7 in]
                n1552 = call-dynamic "Write Comments.vi"("error in (no error)"=w3497, "Comments"=w3515, "Interface in"=w3508) -> ("error out"=w3498:errorcluster, "Interface out"=w3509:refnum<class "Interface.lvclass">)  [unwired: 7 in]
                n1553 = local read "Exp ch2"() -> (w3492:u32)
                n1554 = call-dynamic "Write DS9.vi"("error in (no error)"=w3498, "DS9"="F", "Interface in"=w3509) -> ("error out"=w3485:errorcluster, "Interface out"=w3487:refnum<class "Interface.lvclass">)  [unwired: 7 in]
                n1555 = call-dynamic "Write Observer.vi"("error in (no error)"=w3485, "Observer"=w3483, "Interface in"=w3487) -> ("error out"=w3484:errorcluster, "Interface out"=w3486:refnum<class "Interface.lvclass">)  [unwired: 7 in]
                n1556 = call-dynamic "Write # Images.vi"("error in (no error)"=w3484, "# Images"=w3492, "Interface in"=w3486) -> ("error out"=w3499:errorcluster, "Interface out"=w3510:refnum<class "Interface.lvclass">)  [unwired: 7 in]
                n1557 = property on="Exposure Time ch2" class="Slide (strict)"("Scale.Maximum"=w3472, "Scale.Minimum"=0.0 ("Scale.Range:Minimum")) -> ()  [unwired: 2 in, 2 out]
                n1558 = property on="Exposure Done ch2" class="Slide (strict)"("Scale.Maximum"=w3492, "Scale.Minimum"=0.0 ("Scale.Range:Minimum")) -> ()  [unwired: 2 in, 2 out]
                n1559 = call-dynamic "Write Interface.vi"("error in (no error)"=w3499, "Interface.lvclass"=w3510, "Channel in"=w3504) -> ("error out"=w3482:errorcluster, "Channel out"=w3481:refnum<class "Channel.lvclass">)  [unwired: 7 in]
                n1560 = call-dynamic "Write ciclos.vi"("error in (no error)"=w3482, "ciclos"=w3480, "Channel in"=w3481) -> ("error out"=w3477:errorcluster, "Channel out"=w3479:refnum<class "Channel.lvclass">)  [unwired: 7 in]
                n1561 = call-dynamic "Write sequencias.vi"("error in (no error)"=w3477, "sequencias"=w3475, "Channel in"=w3479) -> ("error out"=w3476:errorcluster, "Channel out"=w3478:refnum<class "Channel.lvclass">)  [unwired: 7 in]
                n1562 = call-dynamic "Write Channel.vi"("error in (no error)"=w3476, "Channel.lvclass"=w3478, "Acquisition in"=w3512) -> ("error out"=w3514:errorcluster, "Acquisition out"=w3513:refnum<class "Acquisition.lvclass">)  [unwired: 7 in]
                n1563 = call "Write AcquisitionB.vi"("error in (no error)"=w3514, "Acquisition.lvclass"=w3513, "S4ACS_GUI in"=w3511) -> ("error out"=w3517:errorcluster, "S4ACS_GUI out"=w3518:refnum<class "S4GUI.lvclass">)  [unwired: 7 in]
              }
              frame #2 {
                # "object"
                # "suffix"
                # "obsType"
                n1564 = call-dynamic "Read AcquisitionC.vi"("error in (no error)"=w3578, "S4ACS_GUI in"=w3579) -> ("error out"=w3568:errorcluster, "Acquisition.lvclass"=w3567:refnum<class "Acquisition.lvclass">, "S4ACS_GUI out"=w3557:refnum<class "S4GUI.lvclass">)  [unwired: 7 in]
                n1565 = call-dynamic "Read Channel.vi"("error in (no error)"=w3568, "Acquisition in"=w3567) -> ("error out"=w3565:errorcluster, "Channel.lvclass"=w3566:refnum<class "Channel.lvclass">, "Acquisition out"=w3556:refnum<class "Acquisition.lvclass">)  [unwired: 7 in]
                n1566 = local read "Exptime ch3"() -> (w3531:dbl)
                n1567 = call-dynamic "Read Interface.vi"("error in (no error)"=w3565, "Channel in"=w3566) -> ("error out"=w3574:errorcluster, "Interface.lvclass"=w3563:refnum<class "Interface.lvclass">, "Channel out"=w3564:refnum<class "Channel.lvclass">)  [unwired: 7 in]
                n1568 = call "Write Exposure Time.vi"("error in (no error)"=w3574, "Exposure Time"=w3531, "Interface in"=w3563) -> ("error out"=w3532:errorcluster, "Interface out"=w3533:refnum<class "Interface.lvclass">)  [unwired: 7 in]
                n1569 = case shown="Default" w3530 {
                  tunnel: w3533 -> [w3581 w3586]
                  tunnel: [w3581 w3585] -> w3529
                  tunnel: [w3580 w3584] -> w3528
                  tunnel: w3532 -> [w3580 w3583]
                  tunnel: w3531 -> [_ w3582]
                  frame "ZERO" {
                  }
                  frame Default {
                    n1570 = call-dynamic "Write prev ExpTime.vi"("error in (no error)"=w3583, "prev ExpTime"=w3582, "Interface in"=w3586) -> ("error out"=w3584:errorcluster, "Interface out"=w3585:refnum<class "Interface.lvclass">)  [unwired: 7 in]
                  }
                }
                n1571 = call-dynamic "Write Suffix.vi"("error in (no error)"=w3528, "Suffix"=w3575, "Interface in"=w3529) -> ("error out"=w3573:errorcluster, "Interface out"=w3562:refnum<class "Interface.lvclass">)  [unwired: 7 in]
                n1572 = call-dynamic "Write ObsType.vi"("error in (no error)"=w3573, "ObsType"=w3548, "Interface in"=w3562) -> ("error out"=w3572:errorcluster, "Interface out"=w3561:refnum<class "Interface.lvclass">)  [unwired: 7 in]
                n1573 = call-dynamic "Write Object.vi"("error in (no error)"=w3572, "Object"=w3547, "Interface in"=w3561) -> ("error out"=w3571:errorcluster, "Interface out"=w3560:refnum<class "Interface.lvclass">)  [unwired: 7 in]
                n1574 = call-dynamic "Write Comments.vi"("error in (no error)"=w3571, "Comments"=w3549, "Interface in"=w3560) -> ("error out"=w3570:errorcluster, "Interface out"=w3559:refnum<class "Interface.lvclass">)  [unwired: 7 in]
                n1575 = call-dynamic "Write DS9.vi"("error in (no error)"=w3570, "DS9"="F", "Interface in"=w3559) -> ("error out"=w3544:errorcluster, "Interface out"=w3546:refnum<class "Interface.lvclass">)  [unwired: 7 in]
                n1576 = local read "Exp ch3"() -> (w3552:u32)
                n1577 = property on="Exposure Time ch3" class="Slide (strict)"("Scale.Maximum"=w3531, "Scale.Minimum"=0.0 ("Scale.Range:Minimum")) -> ()  [unwired: 2 in, 2 out]
                n1578 = call-dynamic "Write Observer.vi"("error in (no error)"=w3544, "Observer"=w3542, "Interface in"=w3546) -> ("error out"=w3543:errorcluster, "Interface out"=w3545:refnum<class "Interface.lvclass">)  [unwired: 7 in]
                n1579 = property on="Exposure Done ch3" class="Slide (strict)"("Scale.Maximum"=w3552, "Scale.Minimum"=0.0 ("Scale.Range:Minimum")) -> ()  [unwired: 2 in, 2 out]
                n1580 = call-dynamic "Write # Images.vi"("error in (no error)"=w3543, "# Images"=w3552, "Interface in"=w3545) -> ("error out"=w3569:errorcluster, "Interface out"=w3558:refnum<class "Interface.lvclass">)  [unwired: 7 in]
                n1581 = call-dynamic "Write Interface.vi"("error in (no error)"=w3569, "Interface.lvclass"=w3558, "Channel in"=w3564) -> ("error out"=w3541:errorcluster, "Channel out"=w3540:refnum<class "Channel.lvclass">)  [unwired: 7 in]
                n1582 = call-dynamic "Write ciclos.vi"("error in (no error)"=w3541, "ciclos"=w3539, "Channel in"=w3540) -> ("error out"=w3536:errorcluster, "Channel out"=w3538:refnum<class "Channel.lvclass">)  [unwired: 7 in]
                n1583 = call-dynamic "Write sequencias.vi"("error in (no error)"=w3536, "sequencias"=w3534, "Channel in"=w3538) -> ("error out"=w3535:errorcluster, "Channel out"=w3537:refnum<class "Channel.lvclass">)  [unwired: 7 in]
                n1584 = call-dynamic "Write Channel.vi"("error in (no error)"=w3535, "Channel.lvclass"=w3537, "Acquisition in"=w3556) -> ("error out"=w3554:errorcluster, "Acquisition out"=w3555:refnum<class "Acquisition.lvclass">)  [unwired: 7 in]
                n1585 = call-dynamic "Write AcquisitionC.vi"("error in (no error)"=w3554, "Acquisition.lvclass"=w3555, "S4ACS_GUI in"=w3557) -> ("error out"=w3576:errorcluster, "S4ACS_GUI out"=w3577:refnum<class "S4GUI.lvclass">)  [unwired: 7 in]
              }
              frame #3 {
                # "object"
                # "suffix"
